vi "rs232.vi"() -> ()   [LabVIEW 2016]
uses:
  <vilib>/Instr/_visa.llb/VISA Flush IO Buffer Mask.ctl
  <vilib>/Instr/_visa.llb/VISA Configure Serial Port (Instr).vi
  <vilib>/Waveform/WDTOps.llb/WDT Append Waveforms DBL.vi
panel:
  out "12.86 mmHg or Greater":bool
  out "LabVIEW Version":string
  out "x = y?":bool
  in  "Control PFD Pump":bool
  in  "Control Blood Pump":bool
  in  "Blood Pump Flow Rate (ml/min)":string
  in  "PFD Pump Flow Rate (ml/min)":string
  out "Blood Sensor 1":bool
  out "Blood Sensor 5":bool
  out "Blood Sensor 4":bool
  out "Blood Sensor 3":bool
  out "Blood Sensor 2":bool
  out "Software Version":string
  in  "?":bool
  out "ESTOP Pressed":bool
  out "Blood Sensor 0":bool
  out "Air Bubble Active":bool
  in  "Tab Control":T1(tab)
  in  "Offset 10":dbl
  in  "Offset 9":dbl
  in  "Offset 8":dbl
  in  "Offset 7":dbl
  in  "Offset 6":dbl
  in  "Offset 5":dbl
  in  "Offset 4":dbl
  in  "Offset 3":dbl
  in  "Offset 1":dbl
  in  "Offset 2":dbl
  out "Pressure PFD4 Out":dbl format="%#_5g"
  out "Pressure PFD4 In":dbl format="%#_5g"
  out "Pressure PFD3 Out":dbl format="%#_5g"
  out "Pressure PFD3 In":dbl format="%#_5g"
  out "Pressure PFD2 Out":dbl format="%#_5g"
  out "Pressure PFD2 In":dbl format="%#_5g"
  out "Pressure PFD1 Out":dbl format="%#_5g"
  out "Pressure PFD1 In":dbl format="%#_5g"
  out "?":dynamicdata(graph)
  out "Pressure Blood Out":dbl format="%#_5g"
  out "Pressure Blood In":dbl format="%#_5g"
  in  "Plot Names":string[](array[string])=["First", "Second"]
  out "Data Read Buffer":string
  out "?":dynamicdata(graph)
  out "Blood In - Blood Out":dbl
  out "PFD4 In - PFD4 Out":dbl
  out "PFD2 In - PFD2 Out":dbl
  out "PFD1 In - PFD1 Out":dbl
  out "PFD3 In - PFD3 Out":dbl
  out "?":dynamicdata(graph)
  out "?":dynamicdata(graph)
  out "P1":dbl format="%#_3g"
  out "P2":dbl format="%#_3g"
  out "P3":dbl format="%#_3g"
  out "P4":dbl format="%#_3g"
  out "P5":dbl format="%#_3g"
  out "P6":dbl format="%#_3g"
  out "P7":dbl format="%#_3g"
  out "P8":dbl format="%#_3g"
  out "P10":dbl format="%#_3g"
  out "P9":dbl format="%#_3g"
  out "P1":dbl format="%#_3g"
  out "P 2":dbl format="%#_3g"
  out "P 3":dbl format="%#_3g"
  out "P 4":dbl format="%#_3g"
  out "P 6":dbl format="%#_3g"
  out "P 8":dbl format="%#_3g"
  out "P 10":dbl format="%#_3g"
  out "P 5":dbl format="%#_3g"
  out "P 7":dbl format="%#_3g"
  out "P 9":dbl format="%#_3g"
  out "?":dynamicdata(graph)
  out "Temp. (°C)":dbl format="%#_4g"
  out "SO2 (%)":dbl format="%#_4g"
  out "pH":dbl format="%#_3g"
  out "Liquid Flow PFD4":dbl format="%#_5g"
  out "Liquid Flow PFD3":dbl format="%#_5g"
  out "Liquid Flow PFD2":dbl format="%#_5g"
  out "?":dynamicdata(graph)
  out "Liquid Flow PFD1":dbl format="%#_5g"
  out "Liquid Flow Blood":dbl format="%#_5g"
  in  "LFB Offset":dbl
  in  "LFP Offset 2":dbl
  in  "LFP Offset 3":dbl
  in  "LFP Offset 4":dbl
  in  "LFP Offset 1":dbl
  out "?":dynamicdata(graph)
  out "LF Blood AVG":dbl
  out "LF PFD4 AVG":dbl
  out "LF PFD3 AVG":dbl
  out "LF PFD2 AVG":dbl
  out "LF PFD1 AVG":dbl
  out "Airflow (L/min)":dbl format="%#_3g"
  out "Air Pressure (mmHg)":dbl format="%#_3g"
  out "?":dynamicdata(graph)
  in  "Airflow Offset":dbl
  in  "Air Pressure Offset":dbl
  in  "STOP":bool
  in  "VISA resource name":refnum<visa-resource-name>="COM1"
  # "1. Select the VISA resource name with the right com port number.\n2. Rename the channel names for the pressure waveform chart. \n3. Run Labview (the white right arrow on the toolbar). Turn the enclosure box power on if it is not on. Press the START button. \n4. If required, change the offset values of the Pressures, Pressures Delta, Liq. Flow, and Air.\n5. MUST press the STOP button on the right (NOT the ABORT BUTTON on the toolbar!) \n6. A dialogue box will pop up and ask you if you want to save the data. Select NO.\n7. Do your priming and make a folder on your computer to save data. Then, repeat step 3.\n8. When the test end, MUST press the STOP button (NOT THE ABORT BUTTON!)\n9. The dialogue box will pop up again. Select YES this time if you want to save the data.\n10. Select the filepath and name your file.\n***DON'T PRESS THE ABORT BUTTON BECAUSE DATA WILL BE ERASED IN THE MEMORY BUFFER!*** ABORT ONLY WHEN DATA IS NOT NEEDED!"
  # "Channel Names"
  # "Pressures (mmHg)"
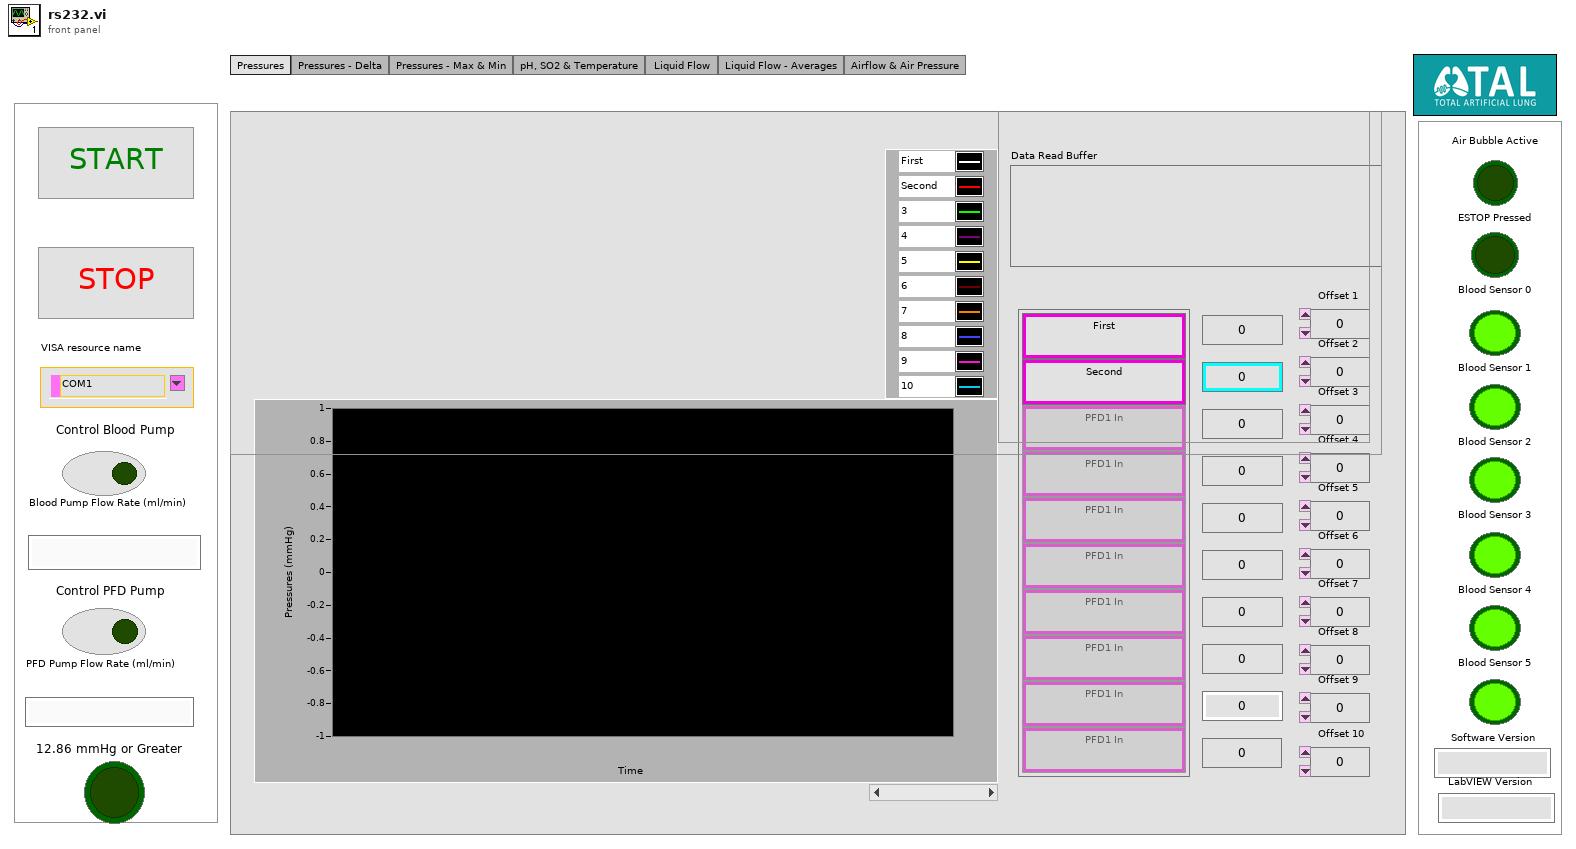
[diagram p1: front panel]
types:
  T1 = enum32{"Pressures", "Pressures - Delta", "Pressures - Max & Min", "pH, SO2 & Temperature", "Liquid Flow ", "Liquid Flow - Averages", "Airflow & Air Pressure"}
  T2 = typedef "VISA Flush IO Buffer Mask.ctl" = u16
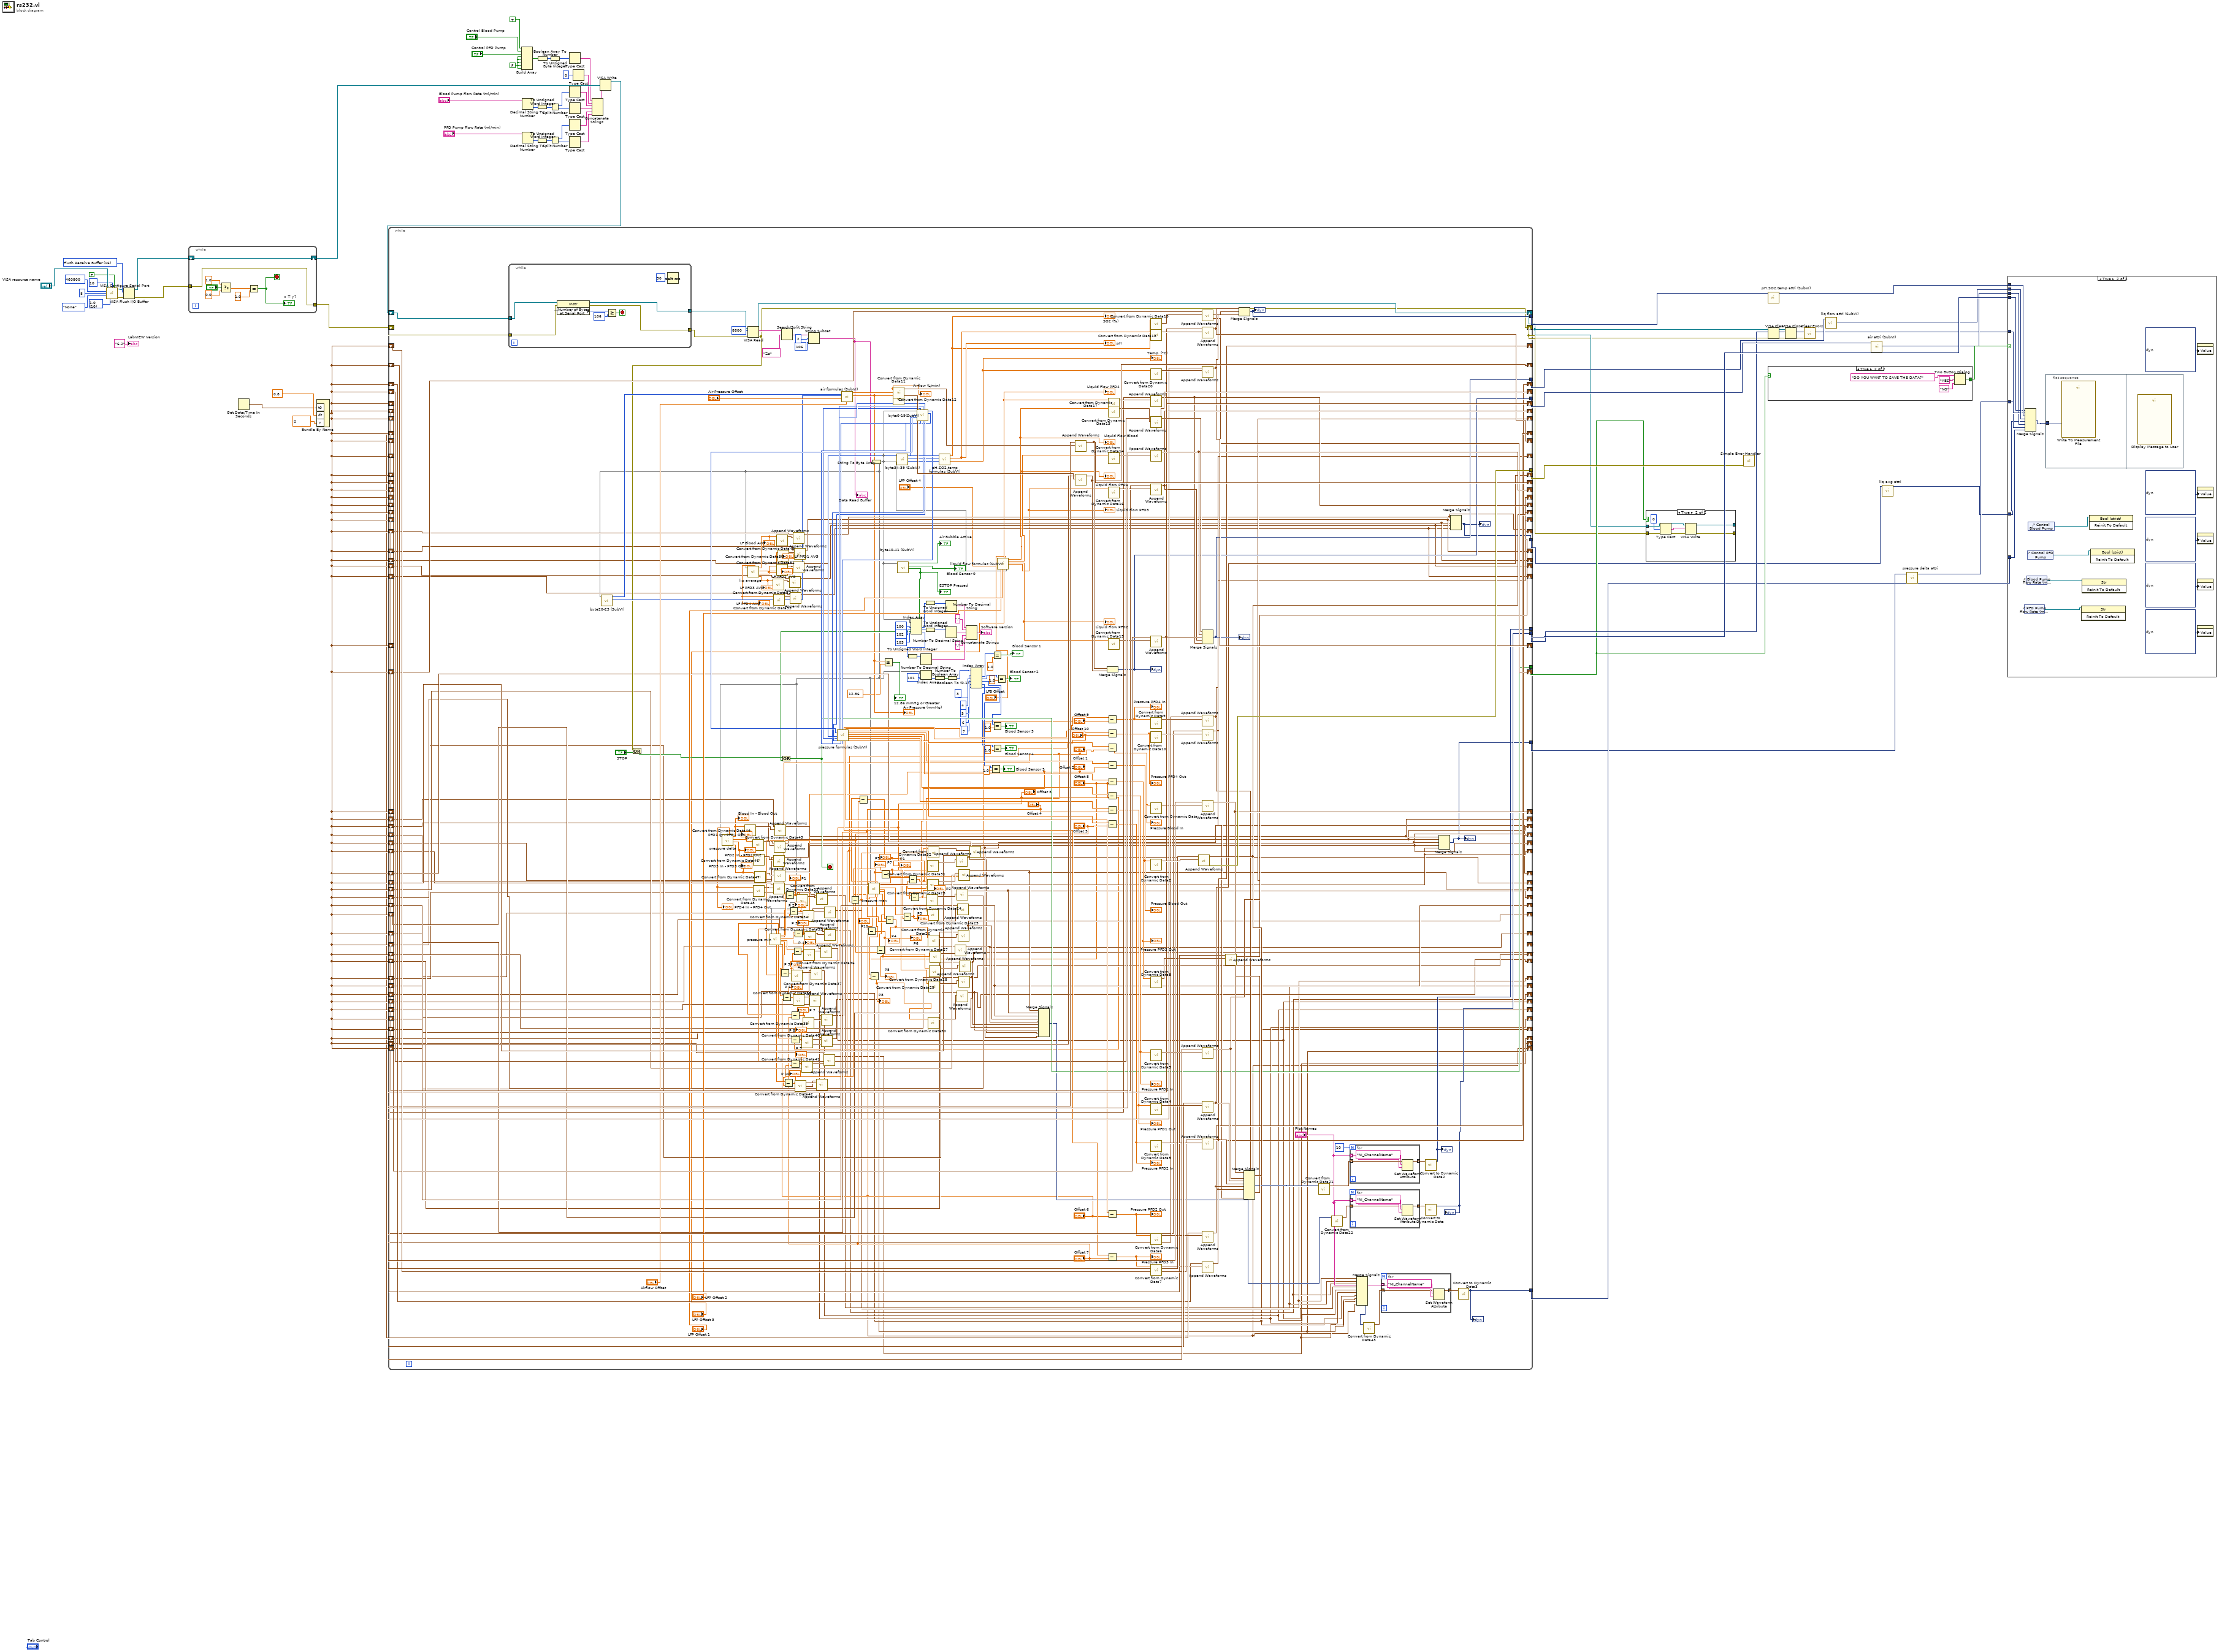
[diagram p0: block diagram]
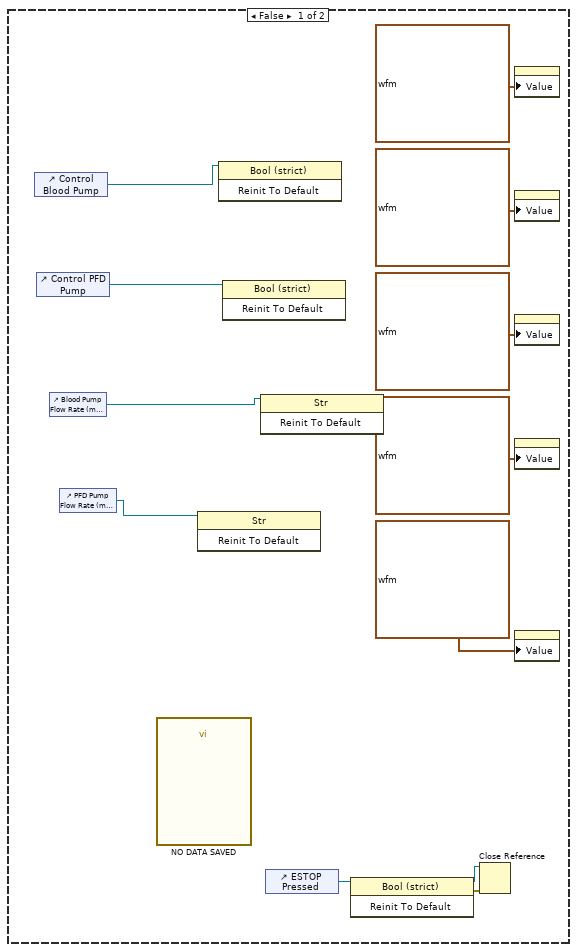
[diagram p3: hidden frame]
diagram:
  w5 = FALSE
  w29 = u16 10 items=["1.0"=10, "1.5"=15, "2.0"=20] ("stop bits (10: 1 bit)")
  w61 = T2 16 items=["Flush Receive Buffer"=16, "Write Transmit Buffer to Device"=32, "Flush Receive Buffer (No I/O)"=64, "Flush Transmit Buffer"=128] ("Mask")
  n1 = call-poly "VISA Configure Serial Port"("VISA resource name"="VISA resource name", "termination char\n(0xA = '\\n' = LF)"=u8 10 ("termination char\n(0xA = '\\n' = LF)"), "Enable Termination\nChar (T)"=FALSE ("Enable Termination\nChar (T)"), "baud rate (9600)"=u32 460800, "data bits (8)"=u16 8, "parity (0:none)"=enum16{"None", "Odd", "Even", "Mark", "Space"}."None", "stop bits (10: 1 bit)"=w29) -> ("VISA resource name out"=w34:refnum<visa-resource-name>, "error out"=w36:errorcluster)  [unwired: 3 in, 4 out]
  n2 = VISA Flush I/O Buffer(VISA resource name=w34, mask (16)=w61, error in (no error)=w36) -> (VISA resource name out=w33:refnum<visa-resource-name>, error out=w35:errorcluster)
  n3 = while {
    tunnel: w35 -> [w68]
    tunnel: [w68] -> w37
    shift-right: [w69] -> w28
    shift-left: w33 -> [w69]
    stop <- w70 stop-if-true
    n4 = Select(t=1.0, s="?", f=0.0) -> (s? t:f=w67:dbl)
    n5 = Equal?(x=w67, y=1.0) -> (x = y?=w70:bool)
    "x = y?" <- w70
  }
  n6 = Get Date/Time In Seconds() -> (seconds since 1Jan1904=w62:timestamp)
  n7 = Bundle By Name("t0"=w62, "dt"=0.8, "Y"=dbl[] []) -> (w40:waveform(dbl))  [unwired: 1 in]
  n8 = Build Array "Build Array"(TRUE, "Control Blood Pump", "Control PFD Pump", w5, w5, w5, w5, w5) -> (w8:bool[])
  n9 = Decimal String To Number(string="Blood Pump Flow Rate (ml/min)") -> (number=w17:i32)  [unwired: 2 in, 1 out]
  n10 = Decimal String To Number(string="PFD Pump Flow Rate (ml/min)") -> (number=w23:i32)  [unwired: 2 in, 1 out]
  n11 = To Unsigned Word Integer(number=w17) -> (unsigned 16bit integer=w16:u16)
  n12 = To Unsigned Word Integer(number=w23) -> (unsigned 16bit integer=w22:u16)
  n13 = Boolean Array To Number(Boolean array=w8) -> (number=w7:u32)
  n14 = To Unsigned Byte Integer(number=w7) -> (unsigned 8bit integer=w9:u8)
  n15 = Split Number(x=w16) -> (hi(x)=w15:u8, lo(x)=w14:u8)
  n16 = Split Number(x=w22) -> (hi(x)=w21:u8, lo(x)=w20:u8)
  n17 = Type Cast(x=w9) -> (*(type *) &x=w10:string)  [unwired: 1 in]
  n18 = Type Cast(x=w15) -> (*(type *) &x=w26:string)  [unwired: 1 in]
  n19 = Type Cast(x=w14) -> (*(type *) &x=w25:string)  [unwired: 1 in]
  n20 = Type Cast(x=w21) -> (*(type *) &x=w24:string)  [unwired: 1 in]
  n21 = Type Cast(x=w20) -> (*(type *) &x=w2:string)  [unwired: 1 in]
  n22 = Type Cast(x=i8 0) -> (*(type *) &x=w11:string)  [unwired: 1 in]
  n23 = Concatenate Strings(w10, w11, w26, w25, w24, w2) -> (w3:string)
  n24 = VISA Write(VISA resource name=w28, write buffer=w3) -> (VISA resource name out=w27:refnum<visa-resource-name>)  [unwired: 1 in, 2 out]
  n25 = while {
    shift-right: [w279] -> w45
    shift-left: w37 -> [w293]
    shift-right: [w314] -> _
    shift-left: w40 -> [w413]
    tunnel: [w416] -> w49
    shift-right: [w313] -> _
    shift-left: w40 -> [w412]
    shift-right: [w312] -> _
    shift-left: w40 -> [w411]
    shift-right: [w311] -> _
    shift-left: w40 -> [w410]
    shift-right: [w310] -> _
    shift-left: w40 -> [w407]
    shift-right: [w309] -> _
    shift-left: w40 -> [w406]
    shift-right: [w308] -> _
    shift-left: w40 -> [w403]
    shift-right: [w307] -> _
    shift-left: w40 -> [w402]
    shift-right: [w306] -> _
    shift-left: w40 -> [w400]
    shift-right: [w305] -> _
    shift-left: w40 -> [w398]
    shift-right: [w393] -> _
    shift-left: w40 -> [w395]
    shift-right: [w392] -> _
    shift-left: w40 -> [w394]
    shift-right: [w387] -> _
    shift-left: w40 -> [w389]
    shift-right: [w386] -> _
    shift-left: w40 -> [w388]
    shift-right: [w379] -> _
    shift-left: w40 -> [w382]
    shift-right: [w378] -> _
    shift-left: w40 -> [w381]
    shift-right: [w377] -> _
    shift-left: w40 -> [w380]
    shift-right: [w372] -> _
    shift-left: w40 -> [w374]
    shift-right: [w323] -> _
    shift-left: w40 -> [w325]
    shift-right: [w371] -> _
    shift-left: w40 -> [w373]
    tunnel: [w304] -> w59
    tunnel: [w317] -> w57
    tunnel: [w316] -> w55
    tunnel: [w315] -> w53
    tunnel: [w281] -> w47
    tunnel: [w301] -> w51
    shift-right: [w295] -> w46
    shift-left: w27 -> [w144]
    shift-right: [w130] -> _
    shift-left: w40 -> [w235]
    shift-right: [w129] -> _
    shift-left: w40 -> [w234]
    shift-right: [w138] -> _
    shift-left: w40 -> [w233]
    shift-right: [w137] -> _
    shift-left: w40 -> [w232]
    shift-right: [w136] -> _
    shift-left: w40 -> [w231]
    shift-right: [w135] -> _
    shift-left: w40 -> [w230]
    shift-right: [w134] -> _
    shift-left: w40 -> [w229]
    shift-right: [w133] -> _
    shift-left: w40 -> [w228]
    shift-right: [w132] -> _
    shift-left: w40 -> [w227]
    shift-right: [w131] -> _
    shift-left: w40 -> [w226]
    shift-right: [w97] -> _
    shift-left: w40 -> [w195]
    shift-right: [w96] -> _
    shift-left: w40 -> [w194]
    shift-right: [w95] -> _
    shift-left: w40 -> [w193]
    shift-right: [w94] -> _
    shift-left: w40 -> [w192]
    shift-right: [w93] -> _
    shift-left: w40 -> [w191]
    shift-right: [w92] -> _
    shift-left: w40 -> [w190]
    shift-right: [w91] -> _
    shift-left: w40 -> [w189]
    shift-right: [w90] -> _
    shift-left: w40 -> [w188]
    shift-right: [w89] -> _
    shift-left: w40 -> [w187]
    shift-right: [w88] -> _
    shift-left: w40 -> [w186]
    tunnel: [w182] -> w43
    shift-right: [w171] -> _
    shift-left: w40 -> [w176]
    shift-right: [w170] -> _
    shift-left: w40 -> [w175]
    shift-right: [w169] -> _
    shift-left: w40 -> [w174]
    shift-right: [w168] -> _
    shift-left: w40 -> [w173]
    shift-right: [w167] -> _
    shift-left: w40 -> [w172]
    tunnel: [w166] -> w42
    shift-right: [w150] -> _
    shift-left: w40 -> [w155]
    shift-right: [w148] -> _
    shift-left: w40 -> [w153]
    shift-right: [w149] -> _
    shift-left: w40 -> [w154]
    shift-right: [w147] -> _
    shift-left: w40 -> [w152]
    shift-right: [w146] -> _
    shift-left: w40 -> [w151]
    tunnel: [w145] -> w39
    stop <- w281 stop-if-true
    n26 = while {
      tunnel: [w435] -> w280
      tunnel: w293 -> [w431]
      tunnel: w144 -> [w430]
      tunnel: [w434] -> w296
      stop <- w436 stop-if-true
      n27 = property class="Instr"(reference=w430, error in=w431) -> (reference out=w434:refnum<visa-resource-name>, error out=w435:errorcluster, "Serial Settings:Number of Bytes at Serial Port"=w433:u32)
      n28 = Greater Or Equal?(x=w433, y=u32 106) -> (x >= y?=w436:bool)
      n29 = Wait (ms)(milliseconds to wait=u32 50) -> ()  [unwired: 1 out]
    }
    n30 = VISA Read(VISA resource name=w296, byte count=u32 8800, error in (no error)=w280) -> (VISA resource name out=w295:refnum<visa-resource-name>, read buffer=w292:string, error out=w279:errorcluster)  [unwired: 1 out]
    n31 = Or(x=w279, y="STOP") -> (x .or. y?=w282:bool)
    n32 = Search/Split String(string=w292, search string/char (-)="Z¥" ("format string")) -> (match + rest of string=w290:string)  [unwired: 1 in, 2 out]
    n33 = String Subset(string=w290, offset (0)=2, length (rest)=106 ("length (rest)")) -> (substring=w76:string)
    "Data Read Buffer" <- w76
    n34 = String To Byte Array(string=w76) -> (unsigned byte array=w75:u8[])
    n35 = call "byte20-23 (SubVI).vi"("unsigned byte array"=w75) -> ("Numeric"=w328:u16, "Numeric 2"=w337:u16)  [unwired: 9 in]
    n36 = call "pressure delta.vi"("unsigned byte array"=w75) -> ("x-y 4"=w83:dbl, "x-y 3"=w84:dbl, "x-y 2"=w85:dbl, "x-y 1"=w86:dbl, "x-y  5"=w82:dbl)  [unwired: 6 in]
    "Blood In - Blood Out" <- w86
    "PFD1 In - PFD1 Out" <- w85
    "PFD2 In - PFD2 Out" <- w84
    "PFD3 In - PFD3 Out" <- w83
    "PFD4 In - PFD4 Out" <- w82
    n37 = call "Convert from Dynamic Data44"("Dynamic Data Type"=w86) -> ("Waveform"=w181:waveform(dbl))  [unwired: 3 in]
    n38 = call "liq average.vi"("unsigned byte array"=w75) -> ("Numeric 4"=w157:dbl, "Numeric 3"=w158:dbl, "Numeric 2"=w159:dbl, "Numeric"=w164:dbl, "Numeric 5"=w156:dbl)  [unwired: 6 in]
    "LF Blood AVG" <- w164
    "LF PFD1 AVG" <- w159
    "LF PFD2 AVG" <- w158
    "LF PFD3 AVG" <- w157
    "LF PFD4 AVG" <- w156
    n39 = call "Convert from Dynamic Data45"("Dynamic Data Type"=w85) -> ("Waveform"=w180:waveform(dbl))  [unwired: 3 in]
    n40 = call "Convert from Dynamic Data46"("Dynamic Data Type"=w84) -> ("Waveform"=w179:waveform(dbl))  [unwired: 3 in]
    n41 = call "Convert from Dynamic Data48"("Dynamic Data Type"=w82) -> ("Waveform"=w177:waveform(dbl))  [unwired: 3 in]
    n42 = call "Convert from Dynamic Data47"("Dynamic Data Type"=w83) -> ("Waveform"=w178:waveform(dbl))  [unwired: 3 in]
    n43 = call "pressure min.vi"("unsigned byte array"=w75) -> ("x-y 9"=w199:dbl, "x-y 10"=w196:dbl, "x-y 7"=w205:dbl, "x-y 8"=w202:dbl, "x-y 1"=w223:dbl, "x-y 2"=w220:dbl, "x-y 3"=w217:dbl, "x-y 4"=w214:dbl, "x-y 5"=w211:dbl, "x-y 6"=w208:dbl)  [unwired: 9 in]
    n44 = call "Convert from Dynamic Data52"("Dynamic Data Type"=w157) -> ("Waveform"=w161:waveform(dbl))  [unwired: 3 in]
    n45 = call "Convert from Dynamic Data53"("Dynamic Data Type"=w156) -> ("Waveform"=w160:waveform(dbl))  [unwired: 3 in]
    n46 = call-poly <vilib>:"Append Waveforms.vi"("waveform B"=w179, "waveform A"=w174) -> ("waveform out"=w169:waveform(dbl))  [unwired: 8 in, 1 out]
    n47 = call-poly <vilib>:"Append Waveforms.vi"("waveform B"=w177, "waveform A"=w172) -> ("waveform out"=w167:waveform(dbl))  [unwired: 8 in, 1 out]
    n48 = call-poly <vilib>:"Append Waveforms.vi"("waveform B"=w178, "waveform A"=w173) -> ("waveform out"=w168:waveform(dbl))  [unwired: 8 in, 1 out]
    n49 = call-poly <vilib>:"Append Waveforms.vi"("waveform B"=w180, "waveform A"=w175) -> ("waveform out"=w170:waveform(dbl))  [unwired: 8 in, 1 out]
    n50 = call-poly <vilib>:"Append Waveforms.vi"("waveform B"=w181, "waveform A"=w176) -> ("waveform out"=w171:waveform(dbl))  [unwired: 8 in, 1 out]
    n51 = call "Convert from Dynamic Data49"("Dynamic Data Type"=w164) -> ("Waveform"=w165:waveform(dbl))  [unwired: 3 in]
    n52 = call "Convert from Dynamic Data51"("Dynamic Data Type"=w158) -> ("Waveform"=w162:waveform(dbl))  [unwired: 3 in]
    n53 = call "Convert from Dynamic Data50"("Dynamic Data Type"=w159) -> ("Waveform"=w163:waveform(dbl))  [unwired: 3 in]
    n54 = Subtract(x=w211, y="Offset 5") -> (x-y=w212:dbl)
    "P 5" <- w212
    n55 = Subtract(x=w208, y="Offset 6") -> (x-y=w209:dbl)
    "P 6" <- w209
    n56 = Subtract(x=w196, y="Offset 10") -> (x-y=w197:dbl)
    "P 10" <- w197
    n57 = Subtract(x=w223, y="Offset 1") -> (x-y=w224:dbl)
    "P1" <- w224
    n58 = Subtract(x=w220, y="Offset 2") -> (x-y=w221:dbl)
    "P 2" <- w221
    n59 = call-poly <vilib>:"Append Waveforms.vi"("waveform B"=w161, "waveform A"=w152) -> ("waveform out"=w147:waveform(dbl))  [unwired: 8 in, 1 out]
    n60 = call-poly <vilib>:"Append Waveforms.vi"("waveform B"=w160, "waveform A"=w151) -> ("waveform out"=w146:waveform(dbl))  [unwired: 8 in, 1 out]
    n61 = Subtract(x=w205, y="Offset 7") -> (x-y=w206:dbl)
    "P 7" <- w206
    n62 = Subtract(x=w202, y="Offset 8") -> (x-y=w203:dbl)
    "P 8" <- w203
    n63 = call "Convert from Dynamic Data37"("Dynamic Data Type"=w212) -> ("Waveform"=w213:waveform(dbl))  [unwired: 3 in]
    n64 = Subtract(x=w214, y="Offset 4") -> (x-y=w216:dbl)
    "P 4" <- w216
    n65 = call-poly <vilib>:"Append Waveforms.vi"("waveform B"=w165, "waveform A"=w155) -> ("waveform out"=w150:waveform(dbl))  [unwired: 8 in, 1 out]
    n66 = call-poly <vilib>:"Append Waveforms.vi"("waveform B"=w162, "waveform A"=w153) -> ("waveform out"=w148:waveform(dbl))  [unwired: 8 in, 1 out]
    n67 = Subtract(x=w217, y="Offset 3") -> (x-y=w218:dbl)
    "P 3" <- w218
    n68 = call "Convert from Dynamic Data38"("Dynamic Data Type"=w209) -> ("Waveform"=w210:waveform(dbl))  [unwired: 3 in]
    n69 = call-poly <vilib>:"Append Waveforms.vi"("waveform B"=w163, "waveform A"=w154) -> ("waveform out"=w149:waveform(dbl))  [unwired: 8 in, 1 out]
    n70 = call "Convert from Dynamic Data42"("Dynamic Data Type"=w197) -> ("Waveform"=w198:waveform(dbl))  [unwired: 3 in]
    n71 = call "Convert from Dynamic Data33"("Dynamic Data Type"=w224) -> ("Waveform"=w225:waveform(dbl))  [unwired: 3 in]
    n72 = call "Convert from Dynamic Data40"("Dynamic Data Type"=w203) -> ("Waveform"=w204:waveform(dbl))  [unwired: 3 in]
    n73 = call "Convert from Dynamic Data34"("Dynamic Data Type"=w221) -> ("Waveform"=w222:waveform(dbl))  [unwired: 3 in]
    n74 = call "Convert from Dynamic Data39"("Dynamic Data Type"=w206) -> ("Waveform"=w207:waveform(dbl))  [unwired: 3 in]
    n75 = call "Convert from Dynamic Data36"("Dynamic Data Type"=w216) -> ("Waveform"=w215:waveform(dbl))  [unwired: 3 in]
    n76 = call "Convert from Dynamic Data35"("Dynamic Data Type"=w218) -> ("Waveform"=w219:waveform(dbl))  [unwired: 3 in]
    n77 = call-poly <vilib>:"Append Waveforms.vi"("waveform B"=w210, "waveform A"=w190) -> ("waveform out"=w92:waveform(dbl))  [unwired: 8 in, 1 out]
    n78 = call-poly <vilib>:"Append Waveforms.vi"("waveform B"=w213, "waveform A"=w191) -> ("waveform out"=w93:waveform(dbl))  [unwired: 8 in, 1 out]
    n79 = call-poly <vilib>:"Append Waveforms.vi"("waveform B"=w198, "waveform A"=w186) -> ("waveform out"=w88:waveform(dbl))  [unwired: 8 in, 1 out]
    n80 = call-poly <vilib>:"Append Waveforms.vi"("waveform B"=w225, "waveform A"=w195) -> ("waveform out"=w97:waveform(dbl))  [unwired: 8 in, 1 out]
    n81 = call-poly <vilib>:"Append Waveforms.vi"("waveform B"=w215, "waveform A"=w192) -> ("waveform out"=w94:waveform(dbl))  [unwired: 8 in, 1 out]
    n82 = call-poly <vilib>:"Append Waveforms.vi"("waveform B"=w207, "waveform A"=w189) -> ("waveform out"=w91:waveform(dbl))  [unwired: 8 in, 1 out]
    n83 = call-poly <vilib>:"Append Waveforms.vi"("waveform B"=w204, "waveform A"=w188) -> ("waveform out"=w90:waveform(dbl))  [unwired: 8 in, 1 out]
    n84 = call-poly <vilib>:"Append Waveforms.vi"("waveform B"=w222, "waveform A"=w194) -> ("waveform out"=w96:waveform(dbl))  [unwired: 8 in, 1 out]
    n85 = call-poly <vilib>:"Append Waveforms.vi"("waveform B"=w219, "waveform A"=w193) -> ("waveform out"=w95:waveform(dbl))  [unwired: 8 in, 1 out]
    n86 = call "air formulas (SubVI).vi"("Airflow Offset"="Airflow Offset", "Air Pressure Offset"="Air Pressure Offset", "Numeric in"=w328, "Numeric 4"=w337) -> ("Numeric out"=w79:dbl, "Numeric 3"=w330:dbl)  [unwired: 6 in]
    "Airflow (L/min)" <- w330
    "Air Pressure (mmHg)" <- w79
    n87 = call "pressure max.vi"("unsigned byte array"=w75) -> ("x-y 9"=w102:dbl, "x-y 10"=w99:dbl, "x-y 7"=w108:dbl, "x-y 8"=w105:dbl, "x-y 1"=w127:dbl, "x-y 2"=w124:dbl, "x-y 3"=w120:dbl, "x-y 4"=w118:dbl, "x-y 5"=w114:dbl, "x-y 6"=w111:dbl)  [unwired: 9 in]
    n88 = Subtract(x=w199, y=w102) -> (x-y=w200:dbl)
    "P 9" <- w200
    n89 = call "Convert from Dynamic Data41"("Dynamic Data Type"=w200) -> ("Waveform"=w201:waveform(dbl))  [unwired: 3 in]
    n90 = call-poly <vilib>:"Append Waveforms.vi"("waveform B"=w201, "waveform A"=w187) -> ("waveform out"=w89:waveform(dbl))  [unwired: 8 in, 1 out]
    n91 = Subtract(x=w99, y="Offset 10") -> (x-y=w100:dbl)
    "P10" <- w100
    n92 = Subtract(x=w108, y="Offset 7") -> (x-y=w109:dbl)
    "P7" <- w109
    n93 = Subtract(x=w111, y="Offset 6") -> (x-y=w112:dbl)
    "P6" <- w112
    n94 = Subtract(x=w105, y="Offset 8") -> (x-y=w106:dbl)
    "P8" <- w106
    n95 = Subtract(x=w114, y="Offset 5") -> (x-y=w115:dbl)
    "P5" <- w115
    n96 = Subtract(x=w102, y="Offset 9") -> (x-y=w103:dbl)
    "P9" <- w103
    n97 = Greater Or Equal?(x=w79, y=12.86) -> (x >= y?=→"12.86 mmHg or Greater":bool)
    n98 = Subtract(x=w118, y="Offset 4") -> (x-y=w117:dbl)
    "P4" <- w117
    n99 = call "Convert from Dynamic Data11"("Dynamic Data Type"=w330) -> ("Waveform"=w397:waveform(dbl))  [unwired: 3 in]
    n100 = call "Convert from Dynamic Data12"("Dynamic Data Type"=w79) -> ("Waveform"=w396:waveform(dbl))  [unwired: 3 in]
    n101 = call "byte34-39 (SubVI).vi"("unsigned byte array"=w75) -> ("Numeric 2"=w339:u16, "Numeric"=w326:u16, "Numeric 3"=w370:u16)  [unwired: 8 in]
    n102 = call "byte40-41 (SubVI).vi"("unsigned byte array"=w75) -> ("Boolean"=w80:bool, "Boolean 2"=→"Blood Sensor 0":bool, "Boolean 3"=→"Air Bubble Active":bool)  [unwired: 7 in, 1 out]
    "ESTOP Pressed" <- w80
    n103 = Or(x=w282, y=w80) -> (x .or. y?=w281:bool)
    n104 = Subtract(x=w120, y="Offset 3") -> (x-y=w121:dbl)
    "P3" <- w121
    n105 = Subtract(x=w127, y="Offset 1") -> (x-y=w125:dbl)
    "P1" <- w125
    n106 = Subtract(x=w124, y="Offset 2") -> (x-y=w123:dbl)
    "P2" <- w123
    n107 = Index Array(array=w75, index #1=100 ("index"), index #2=102 ("index"), index #3=103 ("index")) -> (element #1=w278:u8, element #2=w276:u8, element #3=w275:u8)
    n108 = To Unsigned Word Integer(number=w275) -> (unsigned 16bit integer=w274:u16)
    n109 = call "byte0-19(SubVI).vi"("unsigned byte array"=w75) -> ("Numeric 2"=w345:u16, "Numeric"=w342:u16, "Numeric 9"=w365:u16, "Numeric 10"=w368:u16, "Numeric 3"=w348:u16, "Numeric 8"=w362:u16, "Numeric 7"=w360:u16, "Numeric 4"=w351:u16, "Numeric 5"=w354:u16, "Numeric 6"=w357:u16)  [unwired: 5 in]
    n110 = call "pressure formulas (SubVI).vi"("Numeric 18"=w365, "Numeric 16"=w362, "Numeric in"=w342, "Numeric 14"=w360, "Numeric 4"=w345, "Numeric 12"=w357, "Numeric 6"=w348, "Numeric 10"=w354, "Numeric 20"=w368, "Numeric 8"=w351) -> ("Numeric 5"=w346:dbl, "Numeric 9"=w352:dbl, "Numeric 3"=w343:dbl, "Numeric 11"=w355:dbl, "Numeric 19"=w366:dbl, "Numeric out"=w340:dbl, "Numeric 7"=w349:dbl, "Numeric 17"=w363:dbl, "Numeric 15"=w361:dbl, "Numeric 13"=w358:dbl)
    n111 = Number To Decimal String(number=w274) -> (decimal integer string=w269:string)  [unwired: 1 in]
    n112 = Index Array(array=w75, index=101) -> (element=w258:u8)
    n113 = To Unsigned Word Integer(number=w278) -> (unsigned 16bit integer=w277:u16)
    n114 = To Unsigned Word Integer(number=w276) -> (unsigned 16bit integer=w273:u16)
    n115 = call "Convert from Dynamic Data24"("Dynamic Data Type"=w123) -> ("Waveform"=w244:waveform(dbl))  [unwired: 3 in]
    n116 = call "Convert from Dynamic Data31"("Dynamic Data Type"=w103) -> ("Waveform"=w237:waveform(dbl))  [unwired: 3 in]
    n117 = call "Convert from Dynamic Data23"("Dynamic Data Type"=w125) -> ("Waveform"=w245:waveform(dbl))  [unwired: 3 in]
    n118 = call "Convert from Dynamic Data25"("Dynamic Data Type"=w121) -> ("Waveform"=w243:waveform(dbl))  [unwired: 3 in]
    n119 = call "Convert from Dynamic Data30"("Dynamic Data Type"=w106) -> ("Waveform"=w238:waveform(dbl))  [unwired: 3 in]
    n120 = call "Convert from Dynamic Data32"("Dynamic Data Type"=w100) -> ("Waveform"=w236:waveform(dbl))  [unwired: 3 in]
    n121 = call "Convert from Dynamic Data26"("Dynamic Data Type"=w117) -> ("Waveform"=w242:waveform(dbl))  [unwired: 3 in]
    n122 = call "Convert from Dynamic Data29"("Dynamic Data Type"=w109) -> ("Waveform"=w239:waveform(dbl))  [unwired: 3 in]
    n123 = call "Convert from Dynamic Data28"("Dynamic Data Type"=w112) -> ("Waveform"=w240:waveform(dbl))  [unwired: 3 in]
    n124 = call "Convert from Dynamic Data27"("Dynamic Data Type"=w115) -> ("Waveform"=w241:waveform(dbl))  [unwired: 3 in]
    n125 = Number To Boolean Array(number=w258) -> (Boolean array=w259:bool[])
    n126 = call "pH,SO2,temp formulas (SubVI).vi"("Numeric 4"=w339, "Numeric in"=w326, "Numeric 6"=w370) -> ("Numeric 3"=w338:dbl, "Numeric 5"=w369:dbl, "Numeric out"=w327:dbl)  [unwired: 6 in]
    "pH" <- w369
    "SO2 (%)" <- w327
    "Temp. (°C)" <- w338
    n127 = Number To Decimal String(number=w277) -> (decimal integer string=w271:string)  [unwired: 1 in]
    n128 = Number To Decimal String(number=w273) -> (decimal integer string=w270:string)  [unwired: 1 in]
    n129 = Boolean To (0,1)(Boolean=w259) -> (0, 1=w260:i16[])
    n130 = call-poly <vilib>:"Append Waveforms.vi"("waveform B"=w241, "waveform A"=w229) -> ("waveform out"=w134:waveform(dbl))  [unwired: 8 in, 1 out]
    n131 = call-poly <vilib>:"Append Waveforms.vi"("waveform B"=w237, "waveform A"=w234) -> ("waveform out"=w129:waveform(dbl))  [unwired: 8 in, 1 out]
    n132 = call-poly <vilib>:"Append Waveforms.vi"("waveform B"=w244, "waveform A"=w232) -> ("waveform out"=w137:waveform(dbl))  [unwired: 8 in, 1 out]
    n133 = call-poly <vilib>:"Append Waveforms.vi"("waveform B"=w238, "waveform A"=w226) -> ("waveform out"=w131:waveform(dbl))  [unwired: 8 in, 1 out]
    n134 = call-poly <vilib>:"Append Waveforms.vi"("waveform B"=w243, "waveform A"=w231) -> ("waveform out"=w136:waveform(dbl))  [unwired: 8 in, 1 out]
    n135 = call-poly <vilib>:"Append Waveforms.vi"("waveform B"=w242, "waveform A"=w230) -> ("waveform out"=w135:waveform(dbl))  [unwired: 8 in, 1 out]
    n136 = call-poly <vilib>:"Append Waveforms.vi"("waveform B"=w239, "waveform A"=w227) -> ("waveform out"=w132:waveform(dbl))  [unwired: 8 in, 1 out]
    n137 = call-poly <vilib>:"Append Waveforms.vi"("waveform B"=w245, "waveform A"=w233) -> ("waveform out"=w138:waveform(dbl))  [unwired: 8 in, 1 out]
    n138 = call-poly <vilib>:"Append Waveforms.vi"("waveform B"=w240, "waveform A"=w228) -> ("waveform out"=w133:waveform(dbl))  [unwired: 8 in, 1 out]
    n139 = Concatenate Strings(w271, "." ("string"), w270, "." ("string"), w269) -> (→"Software Version":string)
    n140 = call-poly <vilib>:"Append Waveforms.vi"("waveform B"=w236, "waveform A"=w235) -> ("waveform out"=w130:waveform(dbl))  [unwired: 8 in, 1 out]
    n141 = Index Array(array=w260, index #1=3 ("index"), index #2=4 ("index"), index #3=5 ("index"), index #4=6 ("index"), index #5=7 ("index")) -> (element #1=w81:i16, element #2=w266:i16, element #3=w268:i16, element #4=w247:i16, element #5=w246:i16)
    n142 = Equal?(x=w246, y=1.0) -> (x = y?=→"Blood Sensor 5":bool)
    n143 = Equal?(x=w81, y=1.0) -> (x = y?=→"Blood Sensor 1":bool)
    n144 = Equal?(x=w268, y=1.0) -> (x = y?=→"Blood Sensor 3":bool)
    n145 = Equal?(x=w247, y=1.0) -> (x = y?=→"Blood Sensor 4":bool)
    n146 = Equal?(x=w266, y=1.0) -> (x = y?=→"Blood Sensor 2":bool)
    n147 = call "liquid flow formulas (SubVI).vi"("LFP Offset 4"="LFP Offset 4", "LFP Offset in"="LFP Offset 2", "LFP Offset 1"="LFP Offset 1", "LFP Offset 3"="LFP Offset 3", "LFB Offset"="LFB Offset", "unsigned byte array"=w75) -> ("Numeric"=w141:dbl, "Numeric 5"=w336:dbl, "Numeric 4"=w334:dbl, "Numeric 3"=w332:dbl, "Numeric 2"=w142:dbl)  [unwired: 9 in]
    "Liquid Flow Blood" <- w336
    "Liquid Flow PFD1" <- w334
    "Liquid Flow PFD2" <- w332
    "Liquid Flow PFD3" <- w142
    "Liquid Flow PFD4" <- w141
    n148 = Merge Signals(w138, w137, w136, w135, w134, w133, w132, w131, w129, w130) -> (w128:dynamicdata)
    n149 = call-poly <vilib>:"Append Waveforms.vi"("waveform B"=w397, "waveform A"=w395) -> ("waveform out"=w393:waveform(dbl))  [unwired: 8 in, 1 out]
    n150 = call-poly <vilib>:"Append Waveforms.vi"("waveform B"=w396, "waveform A"=w394) -> ("waveform out"=w392:waveform(dbl))  [unwired: 8 in, 1 out]
    n151 = Subtract(x=w346, y="Offset 9") -> (x-y=w344:dbl)
    "Pressure PFD4 In" <- w344
    n152 = Subtract(x=w343, y="Offset 10") -> (x-y=w341:dbl)
    "Pressure PFD4 Out" <- w341
    n153 = Subtract(x=w366, y="Offset 1") -> (x-y=w364:dbl)
    "Pressure Blood In" <- w364
    n154 = Subtract(x=w340, y="Offset 2") -> (x-y=w367:dbl)
    "Pressure Blood Out" <- w367
    n155 = Subtract(x=w349, y="Offset 8") -> (x-y=w347:dbl)
    "Pressure PFD3 Out" <- w347
    n156 = Subtract(x=w363, y="Offset 3") -> (x-y=w322:dbl)
    "Pressure PFD1 In" <- w322
    n157 = Subtract(x=w361, y="Offset 4") -> (x-y=w359:dbl)
    "Pressure PFD1 Out" <- w359
    n158 = Subtract(x=w358, y="Offset 5") -> (x-y=w356:dbl)
    "Pressure PFD2 In" <- w356
    n159 = Subtract(x=w355, y="Offset 6") -> (x-y=w353:dbl)
    "Pressure PFD2 Out" <- w353
    n160 = Subtract(x=w352, y="Offset 7") -> (x-y=w350:dbl)
    "Pressure PFD3 In" <- w350
    n161 = Merge Signals(w393, w392) -> (w315:dynamicdata)
    "?" <- w315
    n162 = call "Convert from Dynamic Data17"("Dynamic Data Type"=w141) -> ("Waveform"=w383:waveform(dbl))  [unwired: 3 in]
    n163 = call "Convert from Dynamic Data13"("Dynamic Data Type"=w336) -> ("Waveform"=w391:waveform(dbl))  [unwired: 3 in]
    n164 = call "Convert from Dynamic Data14"("Dynamic Data Type"=w334) -> ("Waveform"=w390:waveform(dbl))  [unwired: 3 in]
    n165 = call "Convert from Dynamic Data16"("Dynamic Data Type"=w142) -> ("Waveform"=w384:waveform(dbl))  [unwired: 3 in]
    n166 = call "Convert from Dynamic Data15"("Dynamic Data Type"=w332) -> ("Waveform"=w385:waveform(dbl))  [unwired: 3 in]
    n167 = call "Convert from Dynamic Data19"("Dynamic Data Type"=w327) -> ("Waveform"=w324:waveform(dbl))  [unwired: 3 in]
    n168 = call "Convert from Dynamic Data18"("Dynamic Data Type"=w369) -> ("Waveform"=w375:waveform(dbl))  [unwired: 3 in]
    n169 = call "Convert from Dynamic Data20"("Dynamic Data Type"=w338) -> ("Waveform"=w376:waveform(dbl))  [unwired: 3 in]
    n170 = call-poly <vilib>:"Append Waveforms.vi"("waveform B"=w383, "waveform A"=w380) -> ("waveform out"=w377:waveform(dbl))  [unwired: 8 in, 1 out]
    n171 = call-poly <vilib>:"Append Waveforms.vi"("waveform B"=w391, "waveform A"=w389) -> ("waveform out"=w387:waveform(dbl))  [unwired: 8 in, 1 out]
    n172 = call-poly <vilib>:"Append Waveforms.vi"("waveform B"=w390, "waveform A"=w388) -> ("waveform out"=w386:waveform(dbl))  [unwired: 8 in, 1 out]
    n173 = call-poly <vilib>:"Append Waveforms.vi"("waveform B"=w384, "waveform A"=w381) -> ("waveform out"=w378:waveform(dbl))  [unwired: 8 in, 1 out]
    n174 = call-poly <vilib>:"Append Waveforms.vi"("waveform B"=w385, "waveform A"=w382) -> ("waveform out"=w379:waveform(dbl))  [unwired: 8 in, 1 out]
    n175 = call "Convert from Dynamic Data9"("Dynamic Data Type"=w344) -> ("Waveform"=w401:waveform(dbl))  [unwired: 3 in]
    n176 = call "Convert from Dynamic Data10"("Dynamic Data Type"=w341) -> ("Waveform"=w399:waveform(dbl))  [unwired: 3 in]
    n177 = call "Convert from Dynamic Data"("Dynamic Data Type"=w364) -> ("Waveform"=w321:waveform(dbl))  [unwired: 3 in]
    n178 = call "Convert from Dynamic Data2"("Dynamic Data Type"=w367) -> ("Waveform"=w417:waveform(dbl))  [unwired: 3 in]
    n179 = call "Convert from Dynamic Data8"("Dynamic Data Type"=w347) -> ("Waveform"=w404:waveform(dbl))  [unwired: 3 in]
    n180 = call "Convert from Dynamic Data3"("Dynamic Data Type"=w322) -> ("Waveform"=w415:waveform(dbl))  [unwired: 3 in]
    n181 = call "Convert from Dynamic Data4"("Dynamic Data Type"=w359) -> ("Waveform"=w414:waveform(dbl))  [unwired: 3 in]
    n182 = call "Convert from Dynamic Data5"("Dynamic Data Type"=w356) -> ("Waveform"=w409:waveform(dbl))  [unwired: 3 in]
    n183 = call "Convert from Dynamic Data6"("Dynamic Data Type"=w353) -> ("Waveform"=w408:waveform(dbl))  [unwired: 3 in]
    n184 = call "Convert from Dynamic Data7"("Dynamic Data Type"=w350) -> ("Waveform"=w405:waveform(dbl))  [unwired: 3 in]
    n185 = call-poly <vilib>:"Append Waveforms.vi"("waveform B"=w417, "waveform A"=w412) -> ("error out"=w416:errorcluster, "waveform out"=w313:waveform(dbl))  [unwired: 8 in]
    n186 = call-poly <vilib>:"Append Waveforms.vi"("waveform B"=w324, "waveform A"=w325) -> ("waveform out"=w323:waveform(dbl))  [unwired: 8 in, 1 out]
    n187 = call-poly <vilib>:"Append Waveforms.vi"("waveform B"=w375, "waveform A"=w374) -> ("waveform out"=w372:waveform(dbl))  [unwired: 8 in, 1 out]
    n188 = call-poly <vilib>:"Append Waveforms.vi"("waveform B"=w376, "waveform A"=w373) -> ("waveform out"=w371:waveform(dbl))  [unwired: 8 in, 1 out]
    n189 = Merge Signals(w387, w386, w379, w378, w377) -> (w316:dynamicdata)
    "?" <- w316
    n190 = call-poly <vilib>:"Append Waveforms.vi"("waveform B"=w401, "waveform A"=w400) -> ("waveform out"=w306:waveform(dbl))  [unwired: 8 in, 1 out]
    n191 = call-poly <vilib>:"Append Waveforms.vi"("waveform B"=w399, "waveform A"=w398) -> ("waveform out"=w305:waveform(dbl))  [unwired: 8 in, 1 out]
    n192 = call-poly <vilib>:"Append Waveforms.vi"("waveform B"=w321, "waveform A"=w413) -> ("waveform out"=w314:waveform(dbl))  [unwired: 8 in, 1 out]
    n193 = call-poly <vilib>:"Append Waveforms.vi"("waveform B"=w415, "waveform A"=w411) -> ("waveform out"=w312:waveform(dbl))  [unwired: 8 in, 1 out]
    n194 = call-poly <vilib>:"Append Waveforms.vi"("waveform B"=w414, "waveform A"=w410) -> ("waveform out"=w311:waveform(dbl))  [unwired: 8 in, 1 out]
    n195 = call-poly <vilib>:"Append Waveforms.vi"("waveform B"=w409, "waveform A"=w407) -> ("waveform out"=w310:waveform(dbl))  [unwired: 8 in, 1 out]
    n196 = call-poly <vilib>:"Append Waveforms.vi"("waveform B"=w408, "waveform A"=w406) -> ("waveform out"=w309:waveform(dbl))  [unwired: 8 in, 1 out]
    n197 = call-poly <vilib>:"Append Waveforms.vi"("waveform B"=w405, "waveform A"=w403) -> ("waveform out"=w308:waveform(dbl))  [unwired: 8 in, 1 out]
    n198 = call-poly <vilib>:"Append Waveforms.vi"("waveform B"=w404, "waveform A"=w402) -> ("waveform out"=w307:waveform(dbl))  [unwired: 8 in, 1 out]
    n199 = Merge Signals(w372, w323, w371) -> (w317:dynamicdata)
    "?" <- w317
    n200 = Merge Signals(w314, w313, w312, w311, w310, w309, w308, w307, w306, w305) -> (w300:dynamicdata)
    n201 = call "Convert from Dynamic Data21"("Dynamic Data Type"=w300) -> ("Array of Waveform"=w319:waveform(dbl)[])  [unwired: 3 in]
    n202 = call "Convert from Dynamic Data22"("Dynamic Data Type"=w128) -> ("Array of Waveform"=w303:waveform(dbl)[])  [unwired: 3 in]
    n203 = for {
      N: 10 -> [_]
      tunnel: w319 -> [w429] mode=indexing
      tunnel: "Plot Names" -> [w427] mode=indexing
      tunnel: [w426] -> w320 mode=indexing
      n204 = Set Waveform Attribute(5:w427, 6:"NI_ChannelName" ("name"), 7:w429) -> (3:w426:waveform(dbl))  [unwired: 1 in, 2 out]
    }
    n205 = for {
      tunnel: "Plot Names" -> [w424] mode=indexing
      tunnel: w303 -> [w423] mode=indexing
      tunnel: [w422] -> w302 mode=indexing
      n206 = Set Waveform Attribute(5:w424, 6:"NI_ChannelName" ("name"), 7:w423) -> (3:w422:waveform(dbl))  [unwired: 1 in, 2 out]
    }
    n207 = Merge Signals(w97, w96, w95, w94, w93, w92, w91, w90, w89, w88) -> (w87:dynamicdata)
    n208 = call "Convert from Dynamic Data43"("Dynamic Data Type"=w87) -> ("Array of Waveform"=w185:waveform(dbl)[])  [unwired: 3 in]
    n209 = for {
      tunnel: "Plot Names" -> [w420] mode=indexing
      tunnel: w185 -> [w419] mode=indexing
      tunnel: [w418] -> w183 mode=indexing
      n210 = Set Waveform Attribute(5:w420, 6:"NI_ChannelName" ("name"), 7:w419) -> (3:w418:waveform(dbl))  [unwired: 1 in, 2 out]
    }
    n211 = call "Convert to Dynamic Data2"("Array of Waveforms"=w320) -> ("Dynamic Data Type"=w304:dynamicdata)  [unwired: 3 in]
    "?" <- w304
    n212 = call "Convert to Dynamic Data"("Array of Waveforms"=w302) -> ("Dynamic Data Type"=w301:dynamicdata)  [unwired: 3 in]
    "?" <- w301
    n213 = Merge Signals(w171, w170, w169, w168, w167) -> (w166:dynamicdata)
    "?" <- w166
    n214 = Merge Signals(w150, w149, w148, w147, w146) -> (w145:dynamicdata)
    "?" <- w145
    n215 = call "Convert to Dynamic Data3"("Array of Waveforms"=w183) -> ("Dynamic Data Type"=w182:dynamicdata)  [unwired: 3 in]
    "?" <- w182
  }
  n216 = case shown="True" w47 {
    tunnel: w46 -> [_ w443]
    tunnel: w45 -> [_ w442]
    tunnel: [_ w441] -> _
    tunnel: [_ w440] -> _
    frame False {
    }
    frame True {
      n217 = Type Cast(x=i8 0) -> (*(type *) &x=w438:string)  [unwired: 1 in]
      n218 = VISA Write(VISA resource name=w443, write buffer=w438, error in (no error)=w442) -> (VISA resource name out=w441:refnum<visa-resource-name>, error out=w440:errorcluster)  [unwired: 1 out]
    }
  }
  n219 = call <vilib>:"Simple Error Handler.vi"("error in (no error)"=w49) -> ()  [unwired: 4 in, 5 out]
  n220 = call "pH,SO2,temp attri (SubVI).vi"("Dynamic Data"=w57) -> ("Signals Out"=w56:dynamicdata)  [unwired: 10 in]
  n221 = VISA Clear(VISA resource name=w46, error in (no error)=w45) -> (VISA resource name out=w66:refnum<visa-resource-name>, error out=w65:errorcluster)
  n222 = case shown="True" w47 {
    tunnel: [_ w444] -> w58
    frame False {
    }
    frame True {
      n223 = Two Button Dialog(message="DO YOU WANT TO SAVE THE DATA?", 1:"NO" ("F button name (\"Cancel\")"), 2:"YES" ("T button name (\"OK\")")) -> (T button?=w444:bool)
    }
  }
  n224 = VISA Close(VISA resource name=w66, error in (no error)=w65) -> (error out=w50:errorcluster)
  n225 = call <vilib>:"Clear Errors.vi"("error in (no error)"=w50) -> ()  [unwired: 5 in, 2 out]
  n226 = call "liq flow attri (SubVI).vi"("Dynamic Data"=w55) -> ("Signals Out"=w54:dynamicdata)  [unwired: 10 in]
  n227 = call "air attri (SubVI).vi"("Dynamic Data"=w53) -> ("Signals Out"=w52:dynamicdata)  [unwired: 10 in]
  n228 = call "liq avg attri.vi"("Dynamic Data"=w39) -> ("Signals Out"=w38:dynamicdata)  [unwired: 10 in]
  n229 = call "pressure delta attri.vi"("Dynamic Data"=w42) -> ("Signals Out"=w41:dynamicdata)  [unwired: 10 in]
  n230 = case shown="True" w58 {
    tunnel: w59 -> [_ w470]
    tunnel: w56 -> [_ w477]
    tunnel: w54 -> [_ w476]
    tunnel: w52 -> [_ w466]
    tunnel: w51 -> [_ w467]
    tunnel: w43 -> [_ w468]
    tunnel: w41 -> [_ w469]
    tunnel: w38 -> [_ w465]
    frame False {
      n231 = control-ref of="Control Blood Pump"() -> (w448:refnum<vi>)
      n232 = control-ref of="Control PFD Pump"() -> (w449:refnum<vi>)
      n233 = control-ref of="Blood Pump Flow Rate (ml/min)"() -> (w450:refnum<vi>)
      n234 = control-ref of="PFD Pump Flow Rate (ml/min)"() -> (w451:refnum<vi>)
      n235 = call "NO DATA SAVED"() -> ()  [unwired: 10 in, 2 out]
      n236 = invoke class="Str" method="Reinit To Default"(reference=w451) -> ()  [unwired: 2 in, 3 out]
      n237 = invoke class="Bool (strict)" method="Reinit To Default"(reference=w448) -> ()  [unwired: 2 in, 3 out]
      n238 = invoke class="Bool (strict)" method="Reinit To Default"(reference=w449) -> ()  [unwired: 2 in, 3 out]
      n239 = invoke class="Str" method="Reinit To Default"(reference=w450) -> ()  [unwired: 2 in, 3 out]
      n240 = control-ref of="ESTOP Pressed"() -> (w454:refnum<vi>)
      n241 = invoke class="Bool (strict)" method="Reinit To Default"(reference=w454) -> (reference out=w453:refnum<vi>, error out=w452:errorcluster)  [unwired: 2 in, 1 out]
      n242 = Close Reference(reference=w453, error in (no error)=w452) -> ()  [unwired: 1 out]
      n243 = property class="WFChart (strict)"("Value"=waveform(dbl)[] [{"t0"=timestamp(0 s since 1904-01-01), "dt"=1.0, "Y"=[0.0]}]) -> ()  [unwired: 2 in, 2 out]
      n244 = property class="WFChart (strict)"("Value"=waveform(dbl)[] [{"t0"=timestamp(0 s since 1904-01-01), "dt"=1.0, "Y"=[0.0]}]) -> ()  [unwired: 2 in, 2 out]
      n245 = property class="WFChart (strict)"("Value"=waveform(dbl)[] [{"t0"=timestamp(0 s since 1904-01-01), "dt"=1.0, "Y"=[0.0]}]) -> ()  [unwired: 2 in, 2 out]
      n246 = property class="WFChart (strict)"("Value"=waveform(dbl)[] [{"t0"=timestamp(0 s since 1904-01-01), "dt"=1.0, "Y"=[0.0]}]) -> ()  [unwired: 2 in, 2 out]
      n247 = property class="WFChart (strict)"("Value"=waveform(dbl)[] [{"t0"=timestamp(0 s since 1904-01-01), "dt"=1.0, "Y"=[0.0]}]) -> ()  [unwired: 2 in, 2 out]
    }
    frame True {
      n248 = control-ref of="PFD Pump Flow Rate (ml/min)"() -> (w461:refnum<vi>)
      n249 = Merge Signals(w470, w469, w477, w476, w465, w466, w467, w468) -> (w460:dynamicdata)
      n250 = control-ref of="Blood Pump Flow Rate (ml/min)"() -> (w464:refnum<vi>)
      n251 = control-ref of="Control PFD Pump"() -> (w463:refnum<vi>)
      n252 = control-ref of="Control Blood Pump"() -> (w462:refnum<vi>)
      n253 = flat-sequence {
        tunnel: w460 -> [w478]
        frame #0 {
          n254 = call "Write To Measurement File"("Signals"=w478) -> ()  [unwired: 16 in, 3 out]
        }
        frame #1 {
          n255 = call "Display Message to User"() -> ()  [unwired: 10 in, 2 out]
        }
      }
      n256 = invoke class="Str" method="Reinit To Default"(reference=w461) -> ()  [unwired: 2 in, 3 out]
      n257 = invoke class="Str" method="Reinit To Default"(reference=w464) -> ()  [unwired: 2 in, 3 out]
      n258 = invoke class="Bool (strict)" method="Reinit To Default"(reference=w462) -> ()  [unwired: 2 in, 3 out]
      n259 = invoke class="Bool (strict)" method="Reinit To Default"(reference=w463) -> ()  [unwired: 2 in, 3 out]
      n260 = property class="WFChart (strict)"("Value"=dynamicdata [{"t0"=timestamp(0 s since 1904-01-01), "dt"=1.0, "Y"=[0.0]}]) -> ()  [unwired: 2 in, 2 out]
      n261 = property class="WFChart (strict)"("Value"=dynamicdata [{"t0"=timestamp(0 s since 1904-01-01), "dt"=1.0, "Y"=[0.0]}]) -> ()  [unwired: 2 in, 2 out]
      n262 = property class="WFChart (strict)"("Value"=dynamicdata [{"t0"=timestamp(0 s since 1904-01-01), "dt"=1.0, "Y"=[0.0]}]) -> ()  [unwired: 2 in, 2 out]
      n263 = property class="WFChart (strict)"("Value"=dynamicdata [{"t0"=timestamp(0 s since 1904-01-01), "dt"=1.0, "Y"=[0.0]}]) -> ()  [unwired: 2 in, 2 out]
      n264 = property class="WFChart (strict)"("Value"=dynamicdata [{"t0"=timestamp(0 s since 1904-01-01), "dt"=1.0, "Y"=[0.0]}]) -> ()  [unwired: 2 in, 2 out]
    }
  }
  "LabVIEW Version" <- "6.2" ("LabVIEW Version")
